vi "Start Measurement.vi"(8 "error in":errorcluster, 9 "pin map context":T3, 10 "measurement configuration":T1={"ms update interval"=100}, 11 "gRPCid in":T2) -> (0 "error out":errorcluster, 2 "call id":T2, 3 "gRPCid out":T2)   [LabVIEW 2021, in "MeasurementServerTests.lvlib" / "Measurement Service Tests.lvlib" / "Continuous Counting Client.lvlib"]
doc: "Start the measurement for the given measurement configuration."
uses:
  Continuous Counting Client.lvlib
  gRPC/Generated APIs/ni/measurementlink/measurement/v2/Measurement Service Client V2/RPC Messages/ni_measurementlink_PinMapContext.ctl
  <vilib>/gRPC/LabVIEW gRPC Library/Shared/grpcId.ctl
  controls/Measurement Configuration.ctl
  gRPC/Generated APIs/ni/measurementlink/measurement/v2/Measurement Service Client V2/RPC Messages/ni_measurementlink_measurement_v2_MeasureRequest.ctl
  gRPC/Generated APIs/ni/measurementlink/measurement/v2/Measurement Service Client V2/RPC Messages/google_protobuf_Any.ctl
  7061fa50-9f43-4eb3-8fe8-31484f53e761.vi
  <vilib>/gRPC/LabVIEW gRPC Library/Server API/Translate Protobuf Error.vi
  <vilib>/AdvancedString/1D String Array to Delimited String.vi
  <vilib>/gRPC/LabVIEW gRPC Library/Server API/Server/Get Server DLL Path.vi
  gRPC/Generated APIs/ni/measurementlink/measurement/v2/Measurement Service Client V2/Measurement Service Client V2.lvlib
  <vilib>/gRPC/LabVIEW gRPC Library/grpc-lvsupport-release.lvlib
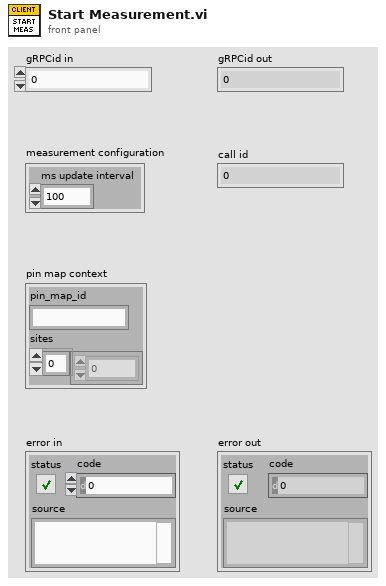
[diagram p1: front panel]
types:
  T1 = typedef "MeasurementServerTests.lvlib/Measurement Service Tests.lvlib/Continuous Counting Client.lvlib/Measurement Configuration.ctl" = cluster{"ms update interval":u32}
  T2 = typedef "grpc-lvsupport-release.lvlib/grpcId.ctl" = u64
  T3 = typedef "Measurement Service Client V2.lvlib/ni_measurementlink_PinMapContext.ctl" = cluster{"pin_map_id":string, "sites":i32[]}
  T4 = typedef "Measurement Service Client V2.lvlib/ni_measurementlink_measurement_v2_MeasureRequest.ctl" = cluster{"configuration_parameters":T5, "pin_map_context":T3}
  T5 = typedef "Measurement Service Client V2.lvlib/google_protobuf_Any.ctl" = cluster{"type_url":string, "value":u8[]}
  T6 = typedef "grpc-lvsupport-release.lvlib/Any.ctl" = cluster{"Type Url":string, "Bytes":u8[]}
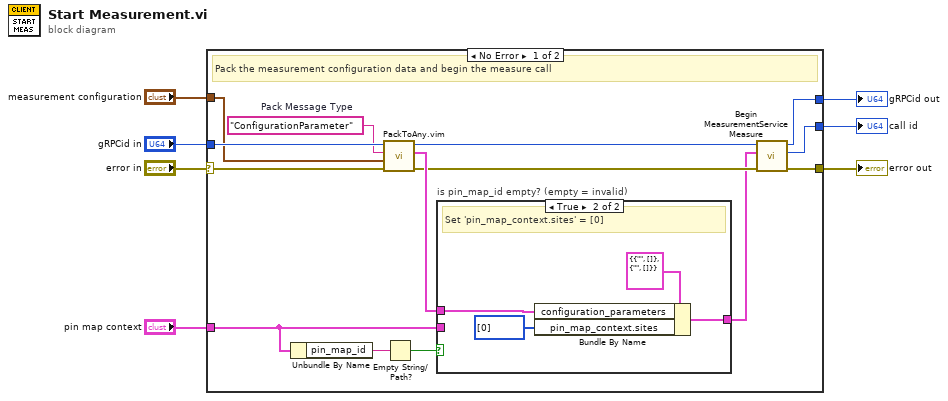
[diagram p0: block diagram]
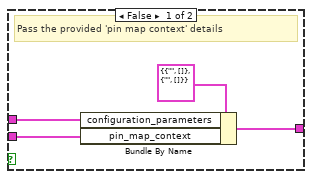
[diagram p2: hidden frame]
diagram:
  n1 = case shown="No Error" "error in" {
    selector: "error in" -> [w18 w30]
    tunnel: "pin map context" -> [w21 _]
    tunnel: "gRPCid in" -> [w19 _]
    tunnel: [w13 w30] -> w4
    tunnel: [w10 _] -> w3
    tunnel: [w11 _] -> w2
    tunnel: "measurement configuration" -> [w16 _]
    frame No Error {
      w17 = "ConfigurationParameter"  # Pack Message Type
      # "Pack the measurement configuration data and begin the measure call"
      n2 = Unbundle By Name(w21) -> ("pin_map_id"=w15:string)
      n3 = call "PackToAny.vim"("error in"=w18, "Data To Pack"=w16, "Message Type"=w17, "gRPCid in"=w19) -> ("error out"=w12:errorcluster, "Any"=w20:T6, "gRPCid out"=w9:u64)  [unwired: 5 in]
      n4 = Empty String/Path?(string/path=w15) -> (empty?=w14:bool)
      n5 = case "is pin_map_id empty? (empty = invalid)" shown="True" w14 {
        tunnel: [w25 w29] -> w8
        tunnel: w21 -> [w24 _]
        tunnel: w20 -> [w23 w28]
        frame False {
          # "Pass the provided 'pin map context' details"
          n6 = Bundle By Name(cluster=T4 {"configuration_parameters"={"type_url"="", "value"=[]}, "pin_map_context"={"pin_map_id"="", "sites"=[]}} ("ni_measurementlink_measurement_v2_MeasureRequest"), "configuration_parameters"=w23, "pin_map_context"=w24) -> (w25:T4)
        }
        frame True {
          # "Set 'pin_map_context.sites' = [0]"
          n7 = Bundle By Name(cluster=T4 {"configuration_parameters"={"type_url"="", "value"=[]}, "pin_map_context"={"pin_map_id"="", "sites"=[]}} ("ni_measurementlink_measurement_v2_MeasureRequest"), "configuration_parameters"=w28, "pin_map_context.sites"=i32[] [0]) -> (w29:T4)
        }
      }
      n8 = call "Begin MeasurementService Measure.vi"("error in"=w12, "Request Data"=w8, "gRPC ID"=w9) -> ("error out"=w13:errorcluster, "Call Id Out"=w10:T2, "gRPC ID out"=w11:T2)  [unwired: 6 in]
    }
    frame Error {
      # "Pass"
    }
  }
  "error out" <- w4
  "call id" <- w3
  "gRPCid out" <- w2
